vi "read.vi"(8 "error in (no error)":errorcluster, 11 "Instrument in":refnum<class "Hardware.lvclass">) -> (0 "error out":errorcluster, 2 "outputs":dbl[](array[numeric]), 3 "Instrument out":refnum<class "Hardware.lvclass">)   [LabVIEW 2017, in "Hardware.lvclass"]
doc: "Read data from the instrument"
uses:
  Hardware.lvclass
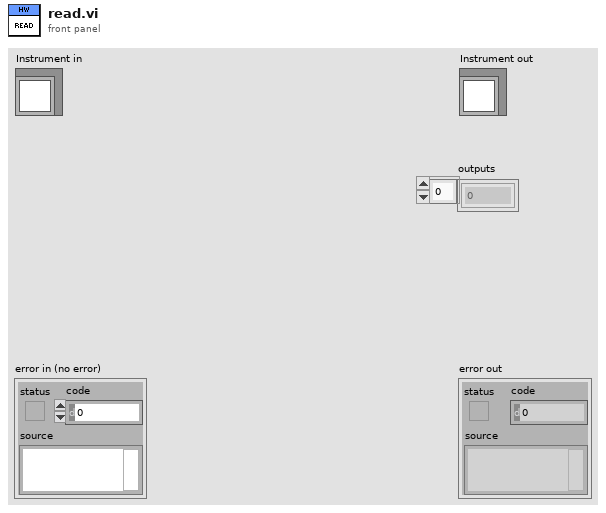
[diagram p1: front panel]
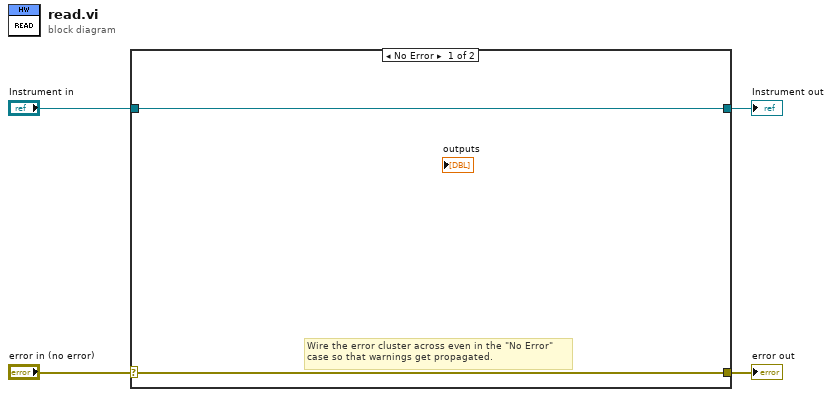
[diagram p0: block diagram]
diagram:
  n1 = case shown="No Error" "error in (no error)" {
    selector: "error in (no error)" -> [w5 w8]
    tunnel: [w5 w8] -> w3
    tunnel: [w6 w7] -> w1
    tunnel: "Instrument in" -> [w6 w7]
    frame No Error {
      # "Wire the error cluster across even in the \"No Error\"\ncase so that warnings get propagated."
    }
    frame Error {
    }
  }
  "error out" <- w3
  "Instrument out" <- w1
